vi "Gui_SetupVoltages.vi"(8 "error in (no error)":errorcluster, 11 "Variant":variant) -> (0 "error out":errorcluster caption="sortie d'erreur", 3 "Variant Output":variant)   [LabVIEW 2015]
uses:
  controls/VOLTAGES_Inputs.ctl
  controls/HEXA_Inputs.ctl
  controls/QUAD_Inputs.ctl
panel:
  in  "Voltages":T1={"Hexa 1"={"Used"=TRUE, "Voltage"=25.0}, "Hexa 2"={"Used"=TRUE, "Voltage"=25.0}, "Hexa 3"={"Used"=TRUE, "Voltage"=25.0}, "Quad 1"={"Used"=TRUE, "Voltage"=25.0}, "Quad 2"={"Used"=TRUE, "Voltage"=25.0}, "Quad 3"={"Used"=TRUE, "Voltage"=25.0}}
  in  "OK":bool
  # "HEXAPOLE"
  # "QUADRIPOLE"
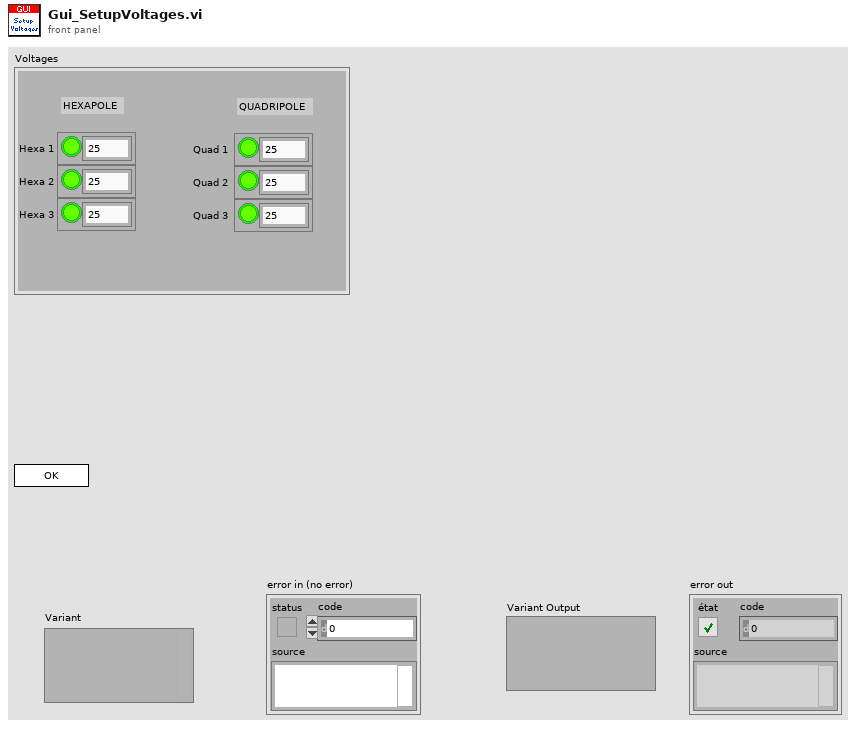
[diagram p1: front panel]
types:
  T1 = typedef "VOLTAGES_Inputs.ctl" = cluster{"Hexa 1":T2, "Hexa 2":T2, "Hexa 3":T2, "Quad 1":T3, "Quad 2":T3, "Quad 3":T3}
  T2 = typedef "HEXA_Inputs.ctl" = cluster{"Used":bool, "Voltage":dbl}
  T3 = typedef "QUAD_Inputs.ctl" = cluster{"Used":bool, "Voltage":dbl}
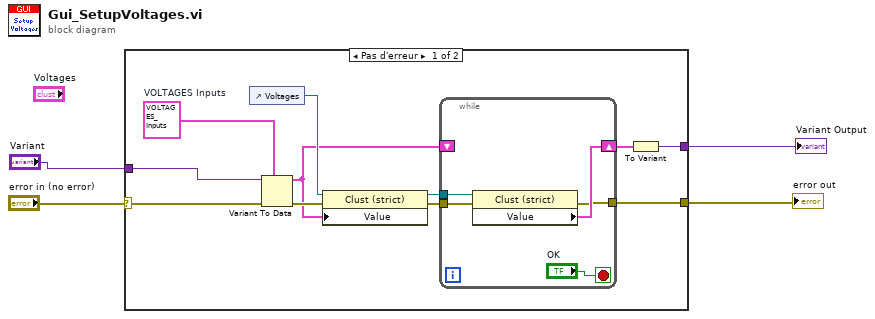
[diagram p0: block diagram]
diagram:
  n1 = case shown="Pas d'erreur" "error in (no error)" {
    selector: "error in (no error)" -> [w13 w22]
    tunnel: [w15 w22] -> w3
    tunnel: [w11 w21] -> w2
    tunnel: "Variant" -> [w9 w21]
    frame No Error {
      w14 = T1 {"Hexa 1"={"Used"=TRUE, "Voltage"=0.0}, "Hexa 2"={"Used"=TRUE, "Voltage"=0.0}, "Hexa 3"={"Used"=TRUE, "Voltage"=0.0}, "Quad 1"={"Used"=TRUE, "Voltage"=25.0}, "Quad 2"={"Used"=TRUE, "Voltage"=25.0}, "Quad 3"={"Used"=TRUE, "Voltage"=25.0}}  # VOLTAGES Inputs
      n2 = control-ref of="Voltages"() -> (w8:refnum<vi>)
      n3 = Variant To Data(error in=w13, type=w14, Variant=w9) -> (data=w7:T1, error out=w10:errorcluster)
      n4 = property class="Clust (strict)"(reference=w8, error in=w10, "Value"=w7) -> (reference out=w6:refnum<vi>, error out=w5:errorcluster)
      n5 = while {
        shift-right: [w18] -> w12
        shift-left: w7 -> [_]
        tunnel: [w16] -> w15
        tunnel: w6 -> [w19]
        tunnel: w5 -> [w17]
        stop <- "OK" stop-if-true
        n6 = property class="Clust (strict)"(reference=w19, error in=w17) -> (error out=w16:errorcluster, "Value"=w18:T1)  [unwired: 1 out]
      }
      n7 = To Variant(anything=w12) -> (Variant=w11:variant)
    }
    frame Error {
    }
  }
  "error out" <- w3
  "Variant Output" <- w2
